vi "TranslatorBooster Build VI Inputs.vi"(8 "error in (no error)":errorcluster, 10 "Function parameters":string[](array[string]), 11 "VI in":refnum<vi>) -> (0 "error out":errorcluster, 2 "ParamsType abbr.":string, 3 "VI out":refnum<vi>)   [LabVIEW 2014, in "Complex Numbers.lvlib"]
uses:
  <vilib>/Aledyne-TSXperts/Arduino Compatible Compiler for LabVIEW/addons/Complex Numbers/Complex Numbers.lvlib
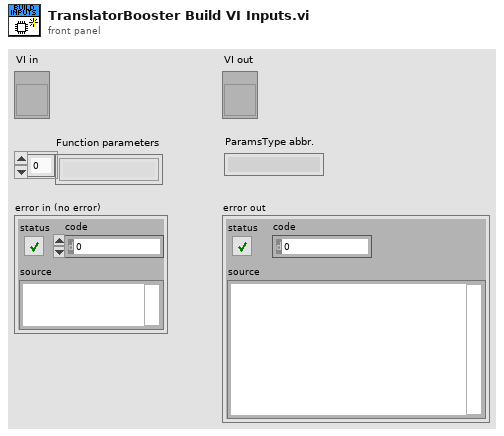
[diagram p1: front panel]
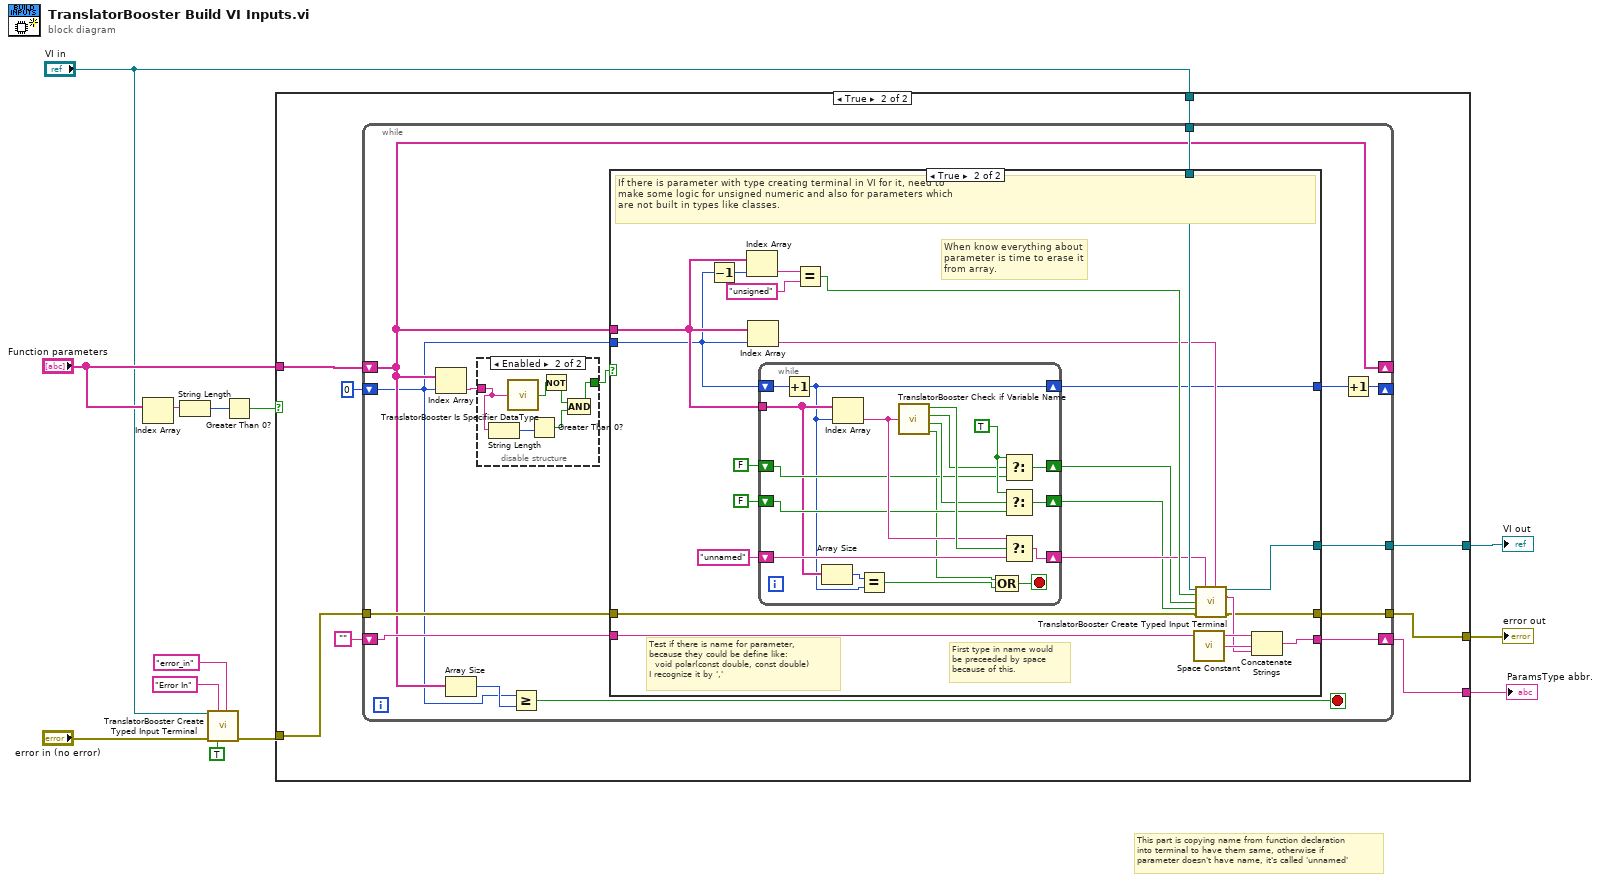
[diagram p0: block diagram]
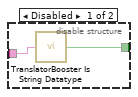
[diagram p3: hidden frame]
diagram:
  # "This part is copying name from function declaration\ninto terminal to have them same, otherwise if\nparameter doesn't have name, it's called 'unnamed'"
  n1 = Index Array(array="Function parameters") -> (element=w9:string)  [unwired: 1 in]
  n2 = String Length(string=w9) -> (length=w8:i32)
  n3 = call <vilib>:"TranslatorBooster Create Typed Input Terminal.vi"("parent VI"="VI in", "Input name"="Error In", "Param type"="error_in", "Error In"="error in (no error)", "Reset?"=TRUE) -> ("Error Out"=w2:errorcluster)  [unwired: 8 in, 2 out]
  n4 = Greater Than 0?(x=w8) -> (x > 0?=w11:bool)
  n5 = case shown="True" w11 {
    tunnel: [w14 w19] -> w13
    tunnel: [w15 w21] -> w12
    tunnel: "Function parameters" -> [_ w23]
    tunnel: w2 -> [w14 w20]
    tunnel: "VI in" -> [w15 w22]
    tunnel: [_ w18] -> w7
    frame False {
    }
    frame True {
      n6 = while {
        tunnel: w22 -> [w36]
        tunnel: [w35] -> w21
        tunnel: w20 -> [w34]
        tunnel: [w33] -> w19
        shift-right: [w28] -> _
        shift-left: w23 -> [w28]
        shift-right: [w30] -> w18
        shift-left: "" -> [w29]
        shift-right: [w24] -> _
        shift-left: 0 -> [w25]
        stop <- w32 stop-if-true
        n7 = Index Array(array=w28, index=w25) -> (element=w37:string)
        n8 = Array Size(array=w28) -> (size(s)=w27:i32)
        n9 = disable-structure shown="Enabled" {
          disable-tunnel: w37 -> [w39 w44]
          disable-tunnel: [w38 w42] -> w31
          frame Disabled {
            n10 = call <vilib>:"TranslatorBooster Is String Datatype.vi"("String token"=w39) -> ("Is datatype?"=w38:bool)
          }
          frame Enabled {
            n11 = String Length(string=w44) -> (length=w40:i32)
            n12 = call <vilib>:"TranslatorBooster Is Specifier DataType.vi"("String token"=w44) -> ("Is specifier?"=w45:bool)
            n13 = Greater Than 0?(x=w40) -> (x > 0?=w41:bool)
            n14 = Not(x=w45) -> (.not. x?=w43:bool)
            n15 = Compound Arithmetic op=AND(w43, w41) -> (w42:bool)
          }
        }
        n16 = Greater Or Equal?(x=w25, y=w27) -> (x >= y?=w32:bool)
        n17 = case shown="True" w31 {
          tunnel: w25 -> [w46 w57]
          tunnel: w36 -> [w48 w61]
          tunnel: [w48 w65] -> w35
          tunnel: w34 -> [w49 w62]
          tunnel: [w49 w63] -> w33
          tunnel: w28 -> [_ w58]
          tunnel: [w47 w68] -> w30
          tunnel: w29 -> [w47 w67]
          tunnel: [w46 w50] -> w26
          frame False {
          }
          frame True {
            # "When know everything about\nparameter is time to erase it\nfrom array."
            # "Test if there is name for parameter,\nbecause they could be define like:\n  void polar(const double, const double)\nI recognize it by ','"
            # "First type in name would\nbe preceeded by space\nbecause of this."
            # "If there is parameter with type creating terminal in VI for it, need to\nmake some logic for unsigned numeric and also for parameters which\nare not built in types like classes."
            n18 = Decrement(x=w57) -> (x-1=w71:i32)
            n19 = Index Array(array=w58, index=w71) -> (element=w70:string)
            n20 = Index Array(array=w58, index=w57) -> (element=w59:string)
            n21 = while {
              tunnel: w58 -> [w78]
              shift-right: [w73] -> w50
              shift-left: w57 -> [w89]
              shift-right: [w86] -> w56
              shift-left: "unnamed" -> [w85]
              shift-right: [w82] -> w54
              shift-left: FALSE -> [w79]
              shift-right: [w81] -> w53
              shift-left: FALSE -> [w80]
              stop <- w74 stop-if-true
              w83 = TRUE
              n22 = Increment(x=w89) -> (x+1=w73:i32)
              n23 = Array Size(array=w78) -> (size(s)=w77:i32)
              n24 = Index Array(array=w78, index=w73) -> (element=w87:string)
              n25 = Equal?(x=w77, y=w73) -> (x = y?=w76:bool)
              n26 = call <vilib>:"TranslatorBooster Check if Variable Name.vi"("String"=w87) -> ("Is Type?"=w88:bool, "Reference?"=w72:bool, "Pointer?"=w84:bool, "Separator?"=w75:bool)  [unwired: 6 in]
              n27 = Compound Arithmetic op=OR(w75, w76) -> (w74:bool)
              n28 = Select(t=w83, s=w72, f=w79) -> (s? t:f=w82:bool)
              n29 = Select(t=w83, s=w84, f=w80) -> (s? t:f=w81:bool)
              n30 = Select(t=w87, s=w88, f=w85) -> (s? t:f=w86:string)
            }
            n31 = Equal?(x=w70, y="unsigned" ("f")) -> (x = y?=w60:bool)
            n32 = call <vilib>:"Space Constant.vi"() -> ("String"=w66:string)
            n33 = call <vilib>:"TranslatorBooster Create Typed Input Terminal.vi"("parent VI"=w61, "Input name"=w56, "Param type"=w59, "Unsigned?"=w60, "Reference?"=w54, "Pointer?"=w53, "Error In"=w62) -> ("parent VI out"=w65:refnum<vi>, "ParamType abbr."=w64:string, "Error Out"=w63:errorcluster)  [unwired: 6 in]
            n34 = Concatenate Strings(w67, w66, w64) -> (w68:string)
          }
        }
        n35 = Increment(x=w26) -> (x+1=w24:i32)
      }
    }
  }
  "error out" <- w13
  "VI out" <- w12
  "ParamsType abbr." <- w7
